vi "Scale Data.vi"(0 "reference in":refnum<class "Adlink.lvclass">, 1 "Raw Data":dbl, 5 "error in (no error)":errorcluster) -> (14 "reference out":refnum<class "Adlink.lvclass">, 15 "Scaled Data":dbl, 19 "error out":errorcluster)   [LabVIEW 2013, in "Adlink.lvclass"]
uses:
  Adlink.lvclass
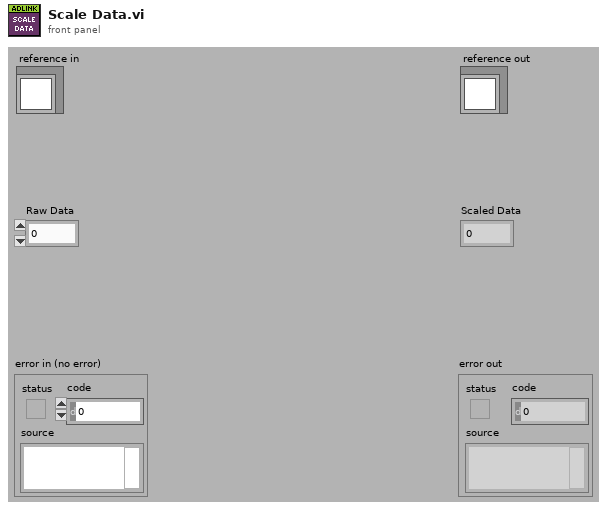
[diagram p1: front panel]
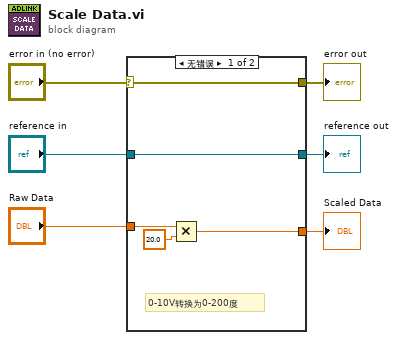
[diagram p0: block diagram]
diagram:
  n1 = case shown="无错误" "error in (no error)" {
    selector: "error in (no error)" -> [w10 w13]
    tunnel: [w10 w13] -> w5
    tunnel: [w11 w12] -> w3
    tunnel: "reference in" -> [w11 w12]
    tunnel: "Raw Data" -> [w9 _]
    tunnel: [w7 _] -> w1
    frame No Error {
      # "0-10V转换为0-200度"
      n2 = Multiply(x=w9, y=20.0) -> (x*y=w7:dbl)
    }
    frame Error {
    }
  }
  "error out" <- w5
  "reference out" <- w3
  "Scaled Data" <- w1
